vi "Server Generate Command Event.vi"(8 "error in":errorcluster, 10 "event data":T1={"client request"={"info data"="", "answer handle"=0}, "command"=enum."Identify"}, 11 "server event ref":refnum<vi>) -> (0 "error out":errorcluster)   [LabVIEW 2018]
doc: "Create server command event."
uses:
  Server Event.ctl
  Server Client Request.ctl
  Server Event Command.ctl
  <vilib>/event_ctls.llb/usereventprio.ctl
  Server Event Ref.ctl
  Server Session.ctl
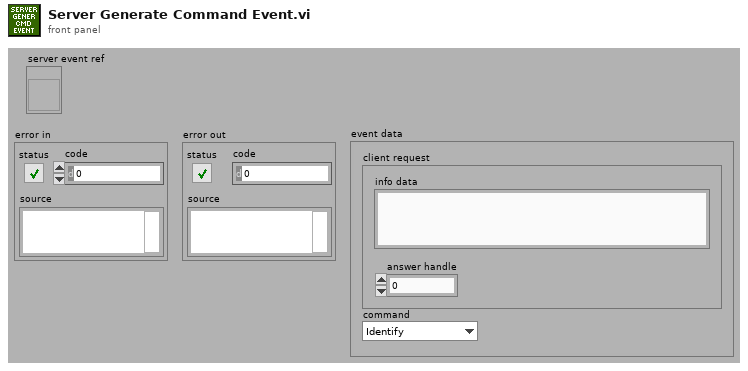
[diagram p1: front panel]
types:
  T1 = typedef "Server Event.ctl" = cluster{"client request":T2, "command":T3}
  T2 = typedef "Server Client Request.ctl" = cluster{"info data":string, "answer handle":i32}
  T3 = typedef "Server Event Command.ctl" = enum16{"None", "Restart", "Identify", "Set measurement", "Start", "Get status", "Get result", "Stop", "Set corrections", "Get algorithm info"}
  T4 = typedef "Server Session.ctl" = cluster{"cmd event":variant, "answer event":variant}
  T5 = typedef "Server Event Ref.ctl" = refnum<user-event>
  T6 = typedef "usereventprio.ctl" = enum32{"high priority", "normal priority"}
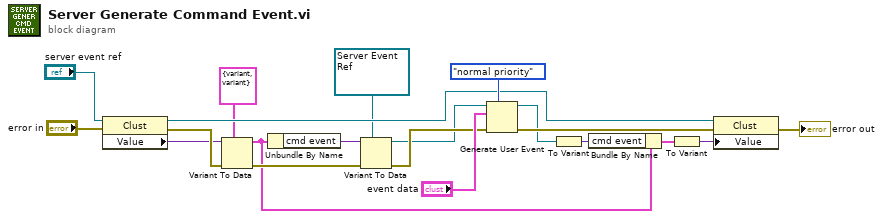
[diagram p0: block diagram]
diagram:
  n1 = property class="Clust"(reference="server event ref", error in="error in") -> (reference out=w16:refnum<vi>, error out=w9:errorcluster, "Value"=w8:variant)
  n2 = Variant To Data(error in=w9, type=T4 {"cmd event"=variant(refnum<user-event> refnum), "answer event"=variant(refnum<user-event> refnum)} ("server"), Variant=w8) -> (data=w3:T4, error out=w7:errorcluster)
  n3 = Unbundle By Name(w3) -> ("cmd event"=w5:variant)
  n4 = Variant To Data(error in=w7, type=T5 refnum ("user event out"), Variant=w5) -> (data=w12:T5, error out=w13:errorcluster)
  n5 = Generate User Event(priority (normal)=usereventprio."normal priority", user event=w12, event data cluster="event data", error in=w13) -> (user event out=w15:T5, error out=w18:errorcluster)
  n6 = To Variant(anything=w15) -> (Variant=w2:variant)
  n7 = Bundle By Name(cluster=w3, "cmd event"=w2) -> (w4:T4)
  n8 = To Variant(anything=w4) -> (Variant=w1:variant)
  n9 = property class="Clust"(reference=w16, error in=w18, "Value"=w1) -> (error out=→"error out":errorcluster)  [unwired: 1 out]
